vi "Autonomous Independent.vi"   [LabVIEW 2020]
doc: "This VI is called when autonomous begins, and will automatically be terminated when autonomous ends. You can carry out timed or sensor driven robot movement independently without needing to return to the caller."
uses:
  <vilib>/Rock Robotics/WPI/Utilities/WPI_GetSetVariantRefNum.vi
  <vilib>/Rock Robotics/Network Tables/NT Read String.vi
  <vilib>/Rock Robotics/Network Tables/NT Write Numeric Array.vi
  Autonomous/AutoGlobals.vi
panel:
  # "Be sure to right-click and choose Data Operations>>Make Current Value default if you want to save the array values with the VI"
types:
  T1 = typedef "WPI_JoystickDevRef.ctl" = cluster{"Device":T2}
  T2 = typedef "WPI_JoystickDeviceEnum.ctl" = enum16{"USB 0", "USB 1", "USB 2", "USB 3", "USB 4", "USB 5"}
  T3 = typedef "Trajectory_Library.lvlib/TRAJECTORY.ctl" = cluster{"TotalTImeSecs":dbl, "States":T4[]}
  T4 = typedef "Trajectory_Library.lvlib/TRAJ_STATE.ctl" = cluster{"TimeSeconds":dbl, "Velocity":dbl, "Acceleration":dbl, "POSE":T5, "Curvature":dbl}
  T5 = typedef "Trajectory_Library.lvlib/POSE2D.ctl" = cluster{"TRANSLATION":T6, "ROTATION":T7}
  T6 = typedef "Trajectory_Library.lvlib/TRANSLATION2D.ctl" = cluster{"X":dbl, "Y":dbl}
  T7 = typedef "Trajectory_Library.lvlib/ROTATION2D.ctl" = cluster{"VALUE":dbl, "COS":dbl, "SIN":dbl}
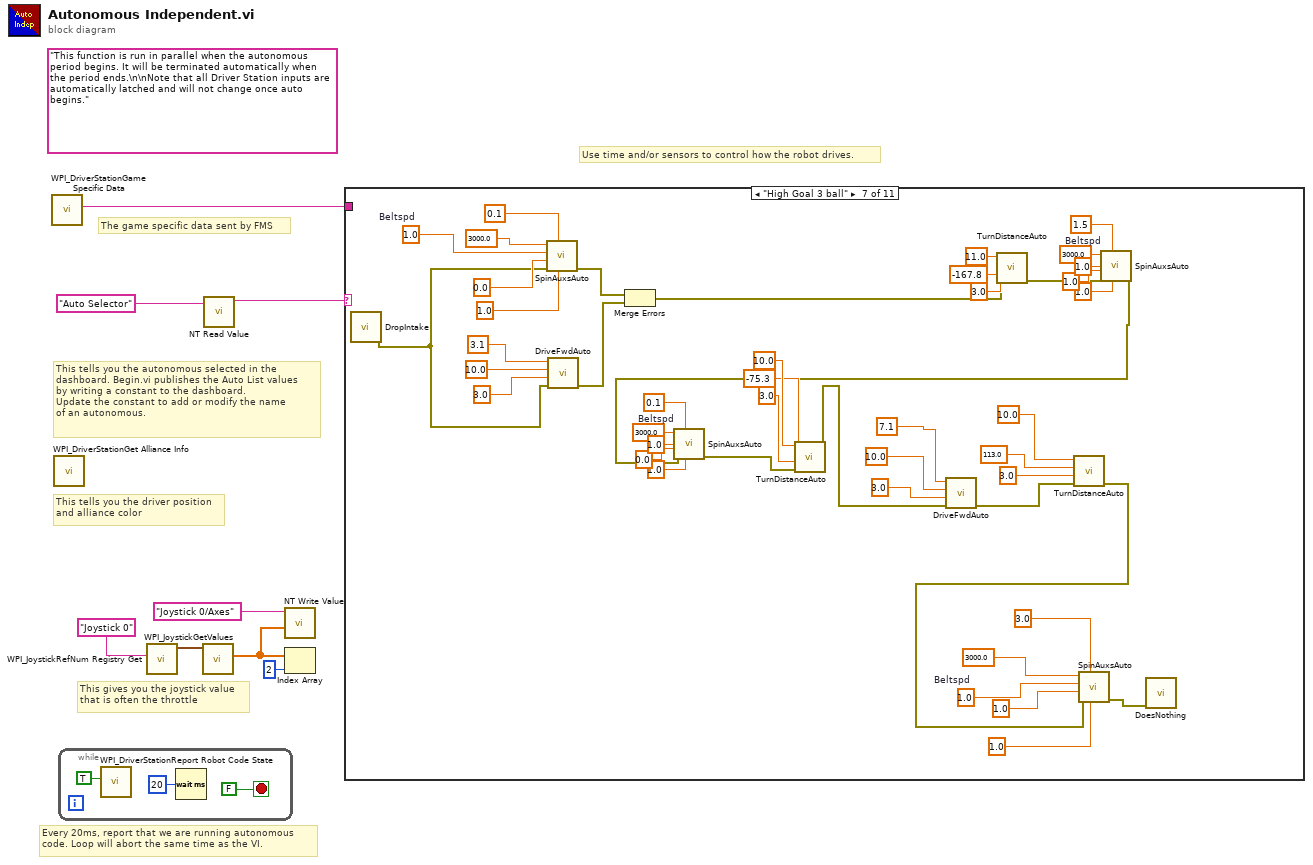
[diagram p0: block diagram]
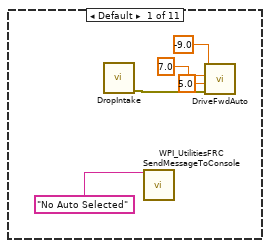
[diagram p2: hidden frame]
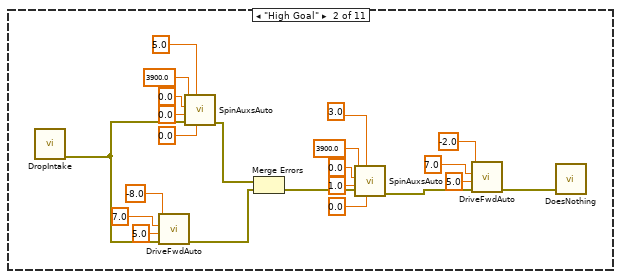
[diagram p3: hidden frame]
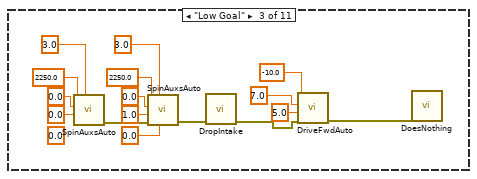
[diagram p4: hidden frame]
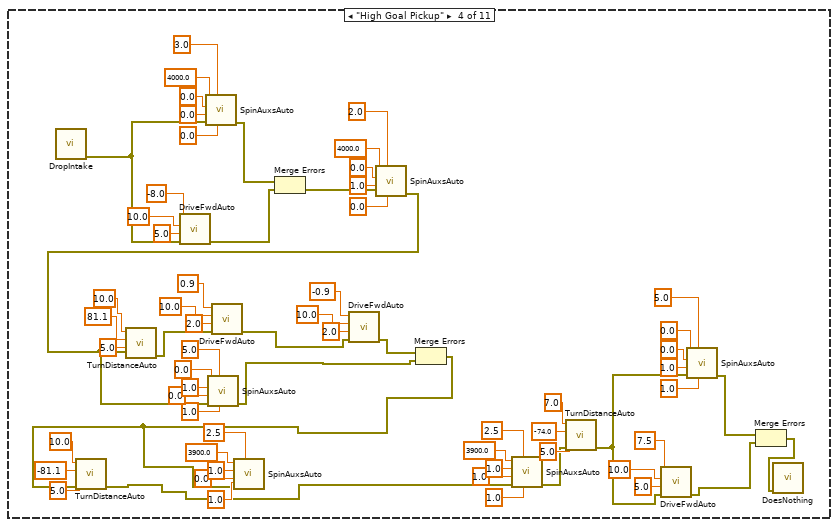
[diagram p5: hidden frame]
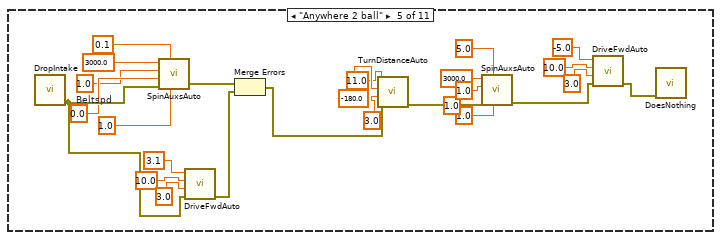
[diagram p6: hidden frame]
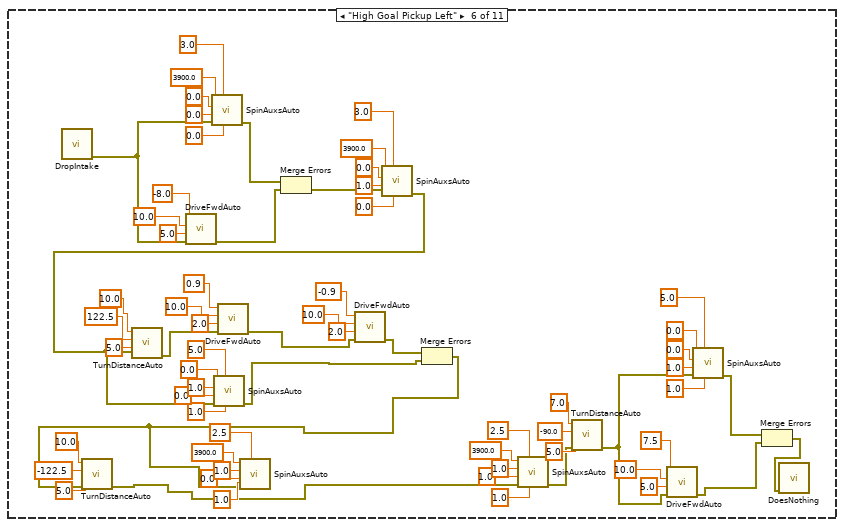
[diagram p7: hidden frame]
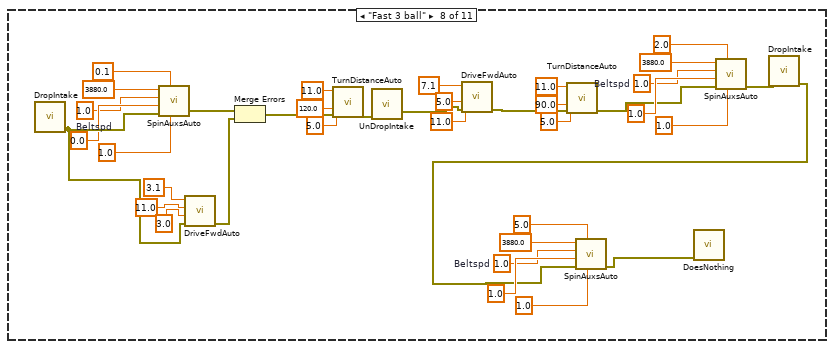
[diagram p8: hidden frame]
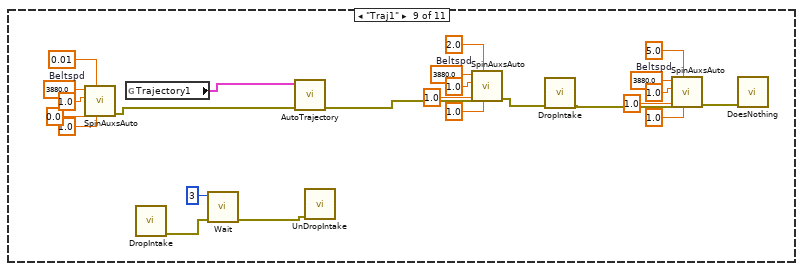
[diagram p9: hidden frame]
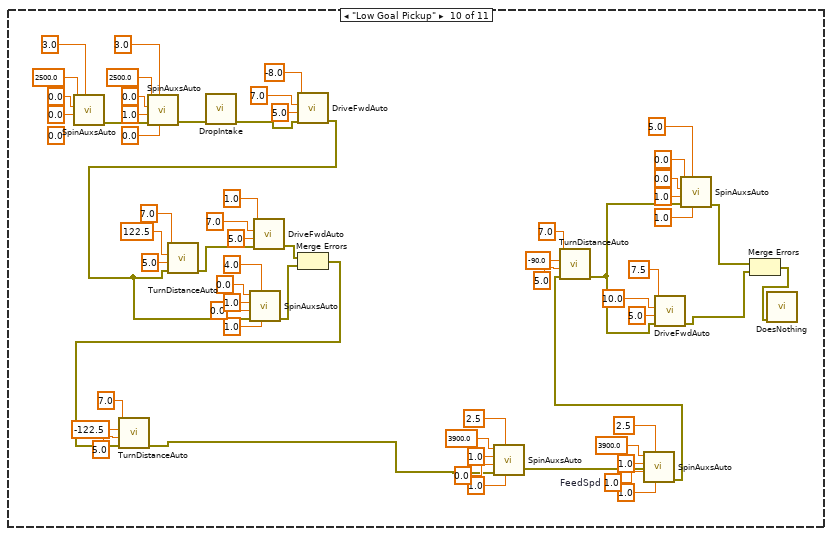
[diagram p10: hidden frame]
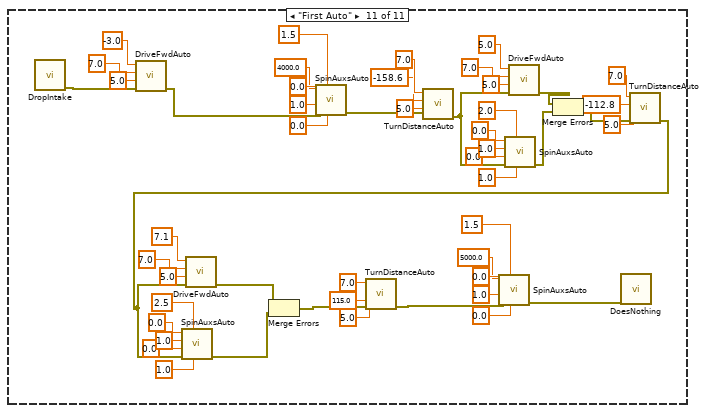
[diagram p11: hidden frame]
diagram:
  (unwired) "This function is run in parallel when the autonomous period begins. It will be terminated automatically when the period ends.\n\nNote that all Driver Station inputs are automatically latched and will not change once auto begins."
  # "The game specific data sent by FMS"
  # "This tells you the autonomous selected in the \ndashboard. Begin.vi publishes the Auto List values\nby writing a constant to the dashboard.\nUpdate the constant to add or modify the name\nof an autonomous."
  # "Every 20ms, report that we are running autonomous\ncode. Loop will abort the same time as the VI."
  # "This gives you the joystick value\nthat is often the throttle"
  # "Use time and/or sensors to control how the robot drives."
  # "This tells you the driver position\nand alliance color"
  n1 = call <vilib>:"WPI_DriverStationGame Specific Data.vi"() -> ("Game Specific Data"=w1:string)  [unwired: 11 in]
  n2 = call <vilib>:"WPI_DriverStationGet Alliance Info.vi"() -> ()  [unwired: 12 out]
  n3 = while {
    stop <- FALSE stop-if-true
    n4 = call <vilib>:"WPI_DriverStationReport Robot Code State.vi"("Autonomous"=TRUE) -> ()  [unwired: 10 in, 1 out]
    n5 = Wait (ms)(milliseconds to wait=u32 20) -> ()  [unwired: 1 out]
  }
  n6 = call <vilib>:"WPI_JoystickRefNum Registry Get.vi"("refnum name"="Joystick 0") -> ("JoystickDevRef"=w7:T1)  [unwired: 1 in, 9 out]
  n7 = call <vilib>:"WPI_JoystickGetValues.vi"("JoystickDevRef"=w7) -> ("Axes"=w3:dbl[])  [unwired: 6 in, 4 out]
  n8 = call-poly <vilib>:"NT Read Value.vi"("Name"="Auto Selector") -> ("String"=w4:string)  [unwired: 9 in, 1 out]
  n9 = call-poly <vilib>:"NT Write Value.vi"("Numeric Array"=w3, "Name"="Joystick 0/Axes") -> ()  [unwired: 9 in, 1 out]
  n10 = Index Array(array=w3, index=2) -> ()  [unwired: 1 out]
  n11 = case shown="\"High Goal 3 ball\"" w4 {
    tunnel: w1 -> [_ _ _ _ _ _ _ _ _ _ _]
    frame Default {
      n12 = call "DropIntake.vi"() -> ("error out"=w13:errorcluster)  [unwired: 11 in]
      n13 = call <vilib>:"WPI_UtilitiesFRC SendMessageToConsole.vi"("Message"="No Auto Selected") -> ()  [unwired: 14 in, 1 out]
      n14 = call "DriveFwdAuto.vi"("error in"=w13, "Timeout"=5.0, "MaxSpeed"=7.0, "Distance"=-9.0) -> ()  [unwired: 6 in, 2 out]
    }
    frame "High Goal" {
      n15 = call "DropIntake.vi"() -> ("error out"=w25:errorcluster)  [unwired: 11 in]
      n16 = call "DriveFwdAuto.vi"("error in"=w25, "Timeout"=5.0, "MaxSpeed"=7.0, "Distance"=-8.0) -> ("error out"=w23:errorcluster)  [unwired: 6 in, 1 out]
      n17 = call "SpinAuxsAuto.vi"("IntakeSpd"=0.0, "Time"=5.0, "error in"=w25, "FeedSpd"=0.0, "Beltspd"=0.0, "ShootSpd"=3900.0) -> ("error out"=w24:errorcluster)  [unwired: 4 in, 1 out]
      n18 = Merge Errors(w24, w23) -> (w22:errorcluster)
      n19 = call "SpinAuxsAuto.vi"("IntakeSpd"=0.0, "Time"=3.0, "error in"=w22, "FeedSpd"=1.0, "Beltspd"=0.0, "ShootSpd"=3900.0) -> ("error out"=w18:errorcluster)  [unwired: 4 in, 1 out]
      n20 = call "DriveFwdAuto.vi"("error in"=w18, "Timeout"=5.0, "MaxSpeed"=7.0, "Distance"=-2.0) -> ("error out"=w17:errorcluster)  [unwired: 6 in, 1 out]
      n21 = call "DoesNothing.vi"("error in (no error)"=w17) -> ()  [unwired: 10 in, 1 out]
    }
    frame "Low Goal" {
      (unwired) 0.0 ("IntakeSpd")
      n22 = call "SpinAuxsAuto.vi"("Time"=3.0, "FeedSpd"=0.0, "Beltspd"=0.0, "ShootSpd"=2250.0) -> ("error out"=w42:errorcluster)  [unwired: 6 in, 1 out]
      n23 = call "SpinAuxsAuto.vi"("IntakeSpd"=0.0, "Time"=3.0, "error in"=w42, "FeedSpd"=1.0, "Beltspd"=0.0, "ShootSpd"=2250.0) -> ("error out"=w41:errorcluster)  [unwired: 4 in, 1 out]
      n24 = call "DropIntake.vi"("error in"=w41) -> ("error out"=w40:errorcluster)  [unwired: 10 in]
      n25 = call "DriveFwdAuto.vi"("error in"=w40, "Timeout"=5.0, "MaxSpeed"=7.0, "Distance"=-10.0) -> ("error out"=w39:errorcluster)  [unwired: 6 in, 1 out]
      n26 = call "DoesNothing.vi"("error in (no error)"=w39) -> ()  [unwired: 10 in, 1 out]
    }
    frame "High Goal Pickup" {
      n27 = call "DropIntake.vi"() -> ("error out"=w118:errorcluster)  [unwired: 11 in]
      n28 = call "DriveFwdAuto.vi"("error in"=w118, "Timeout"=5.0, "MaxSpeed"=10.0, "Distance"=-8.0) -> ("error out"=w120:errorcluster)  [unwired: 6 in, 1 out]
      n29 = call "SpinAuxsAuto.vi"("IntakeSpd"=0.0, "Time"=3.0, "error in"=w118, "FeedSpd"=0.0, "Beltspd"=0.0, "ShootSpd"=4000.0) -> ("error out"=w119:errorcluster)  [unwired: 4 in, 1 out]
      n30 = Merge Errors(w119, w120) -> (w121:errorcluster)
      n31 = call "SpinAuxsAuto.vi"("IntakeSpd"=0.0, "Time"=2.0, "error in"=w121, "FeedSpd"=1.0, "Beltspd"=0.0, "ShootSpd"=4000.0) -> ("error out"=w84:errorcluster)  [unwired: 4 in, 1 out]
      n32 = call "TurnDistanceAuto.vi"("error in"=w84, "Timeout"=5.0, "Degrees"=81.1, "MaxSpeed"=10.0) -> ("error out"=w102:errorcluster)  [unwired: 6 in, 1 out]
      n33 = call "SpinAuxsAuto.vi"("IntakeSpd"=1.0, "Time"=5.0, "error in"=w84, "FeedSpd"=0.0, "Beltspd"=1.0, "ShootSpd"=0.0) -> ("error out"=w79:errorcluster)  [unwired: 4 in, 1 out]
      n34 = call "DriveFwdAuto.vi"("error in"=w102, "Timeout"=2.0, "MaxSpeed"=10.0, "Distance"=0.9) -> ("error out"=w80:errorcluster)  [unwired: 6 in, 1 out]
      n35 = call "DriveFwdAuto.vi"("error in"=w80, "Timeout"=2.0, "MaxSpeed"=10.0, "Distance"=-0.9) -> ("error out"=w78:errorcluster)  [unwired: 6 in, 1 out]
      n36 = Merge Errors(w78, w79) -> (w55:errorcluster)
      n37 = call "TurnDistanceAuto.vi"("error in"=w55, "Timeout"=5.0, "Degrees"=-81.1, "MaxSpeed"=10.0) -> ("error out"=w56:errorcluster)  [unwired: 6 in, 1 out]
      n38 = call "SpinAuxsAuto.vi"("IntakeSpd"=1.0, "Time"=2.5, "error in"=w55, "FeedSpd"=0.0, "Beltspd"=1.0, "ShootSpd"=3900.0) -> ()  [unwired: 4 in, 2 out]
      n39 = call "SpinAuxsAuto.vi"("IntakeSpd"=1.0, "Time"=2.5, "error in"=w56, "FeedSpd"=1.0, "Beltspd"=1.0, "ShootSpd"=3900.0) -> ("error out"=w57:errorcluster)  [unwired: 4 in, 1 out]
      n40 = call "TurnDistanceAuto.vi"("error in"=w57, "Timeout"=5.0, "Degrees"=-74.0, "MaxSpeed"=7.0) -> ("error out"=w66:errorcluster)  [unwired: 6 in, 1 out]
      n41 = call "DriveFwdAuto.vi"("error in"=w66, "Timeout"=5.0, "MaxSpeed"=10.0, "Distance"=7.5) -> ("error out"=w65:errorcluster)  [unwired: 6 in, 1 out]
      n42 = call "SpinAuxsAuto.vi"("IntakeSpd"=1.0, "Time"=5.0, "error in"=w66, "FeedSpd"=1.0, "Beltspd"=0.0, "ShootSpd"=0.0) -> ("error out"=w74:errorcluster)  [unwired: 4 in, 1 out]
      n43 = Merge Errors(w74, w65) -> (w64:errorcluster)
      n44 = call "DoesNothing.vi"("error in (no error)"=w64) -> ()  [unwired: 10 in, 1 out]
    }
    frame "Anywhere 2 ball" {
      w138 = 1.0  # Beltspd
      n45 = call "DropIntake.vi"() -> ("error out"=w145:errorcluster)  [unwired: 11 in]
      n46 = call "SpinAuxsAuto.vi"("IntakeSpd"=1.0, "Time"=0.1, "error in"=w145, "FeedSpd"=0.0, "Beltspd"=w138, "ShootSpd"=3000.0) -> ("error out"=w147:errorcluster)  [unwired: 4 in, 1 out]
      n47 = call "DriveFwdAuto.vi"("error in"=w145, "Timeout"=3.0, "MaxSpeed"=10.0, "Distance"=3.1) -> ("error out"=w146:errorcluster)  [unwired: 6 in, 1 out]
      n48 = Merge Errors(w147, w146) -> (w127:errorcluster)
      n49 = call "TurnDistanceAuto.vi"("error in"=w127, "Timeout"=3.0, "Degrees"=-180.0, "MaxSpeed"=11.0) -> ("error out"=w136:errorcluster)  [unwired: 6 in, 1 out]
      n50 = call "SpinAuxsAuto.vi"("IntakeSpd"=1.0, "Time"=5.0, "error in"=w136, "FeedSpd"=1.0, "Beltspd"=1.0, "ShootSpd"=3000.0) -> ("error out"=w123:errorcluster)  [unwired: 4 in, 1 out]
      n51 = call "DriveFwdAuto.vi"("error in"=w123, "Timeout"=3.0, "MaxSpeed"=10.0, "Distance"=-5.0) -> ("error out"=w122:errorcluster)  [unwired: 6 in, 1 out]
      n52 = call "DoesNothing.vi"("error in (no error)"=w122) -> ()  [unwired: 10 in, 1 out]
    }
    frame "High Goal Pickup Left" {
      n53 = call "DropIntake.vi"() -> ("error out"=w211:errorcluster)  [unwired: 11 in]
      n54 = call "DriveFwdAuto.vi"("error in"=w211, "Timeout"=5.0, "MaxSpeed"=10.0, "Distance"=-8.0) -> ("error out"=w213:errorcluster)  [unwired: 6 in, 1 out]
      n55 = call "SpinAuxsAuto.vi"("IntakeSpd"=0.0, "Time"=3.0, "error in"=w211, "FeedSpd"=0.0, "Beltspd"=0.0, "ShootSpd"=3900.0) -> ("error out"=w212:errorcluster)  [unwired: 4 in, 1 out]
      n56 = Merge Errors(w212, w213) -> (w214:errorcluster)
      n57 = call "SpinAuxsAuto.vi"("IntakeSpd"=0.0, "Time"=3.0, "error in"=w214, "FeedSpd"=1.0, "Beltspd"=0.0, "ShootSpd"=3900.0) -> ("error out"=w177:errorcluster)  [unwired: 4 in, 1 out]
      n58 = call "TurnDistanceAuto.vi"("error in"=w177, "Timeout"=5.0, "Degrees"=122.5, "MaxSpeed"=10.0) -> ("error out"=w195:errorcluster)  [unwired: 6 in, 1 out]
      n59 = call "SpinAuxsAuto.vi"("IntakeSpd"=1.0, "Time"=5.0, "error in"=w177, "FeedSpd"=0.0, "Beltspd"=1.0, "ShootSpd"=0.0) -> ("error out"=w172:errorcluster)  [unwired: 4 in, 1 out]
      n60 = call "DriveFwdAuto.vi"("error in"=w195, "Timeout"=2.0, "MaxSpeed"=10.0, "Distance"=0.9) -> ("error out"=w173:errorcluster)  [unwired: 6 in, 1 out]
      n61 = call "DriveFwdAuto.vi"("error in"=w173, "Timeout"=2.0, "MaxSpeed"=10.0, "Distance"=-0.9) -> ("error out"=w171:errorcluster)  [unwired: 6 in, 1 out]
      n62 = Merge Errors(w171, w172) -> (w148:errorcluster)
      n63 = call "TurnDistanceAuto.vi"("error in"=w148, "Timeout"=5.0, "Degrees"=-122.5, "MaxSpeed"=10.0) -> ("error out"=w149:errorcluster)  [unwired: 6 in, 1 out]
      n64 = call "SpinAuxsAuto.vi"("IntakeSpd"=1.0, "Time"=2.5, "error in"=w148, "FeedSpd"=0.0, "Beltspd"=1.0, "ShootSpd"=3900.0) -> ()  [unwired: 4 in, 2 out]
      n65 = call "SpinAuxsAuto.vi"("IntakeSpd"=1.0, "Time"=2.5, "error in"=w149, "FeedSpd"=1.0, "Beltspd"=1.0, "ShootSpd"=3900.0) -> ("error out"=w150:errorcluster)  [unwired: 4 in, 1 out]
      n66 = call "TurnDistanceAuto.vi"("error in"=w150, "Timeout"=5.0, "Degrees"=-90.0, "MaxSpeed"=7.0) -> ("error out"=w159:errorcluster)  [unwired: 6 in, 1 out]
      n67 = call "DriveFwdAuto.vi"("error in"=w159, "Timeout"=5.0, "MaxSpeed"=10.0, "Distance"=7.5) -> ("error out"=w158:errorcluster)  [unwired: 6 in, 1 out]
      n68 = call "SpinAuxsAuto.vi"("IntakeSpd"=1.0, "Time"=5.0, "error in"=w159, "FeedSpd"=1.0, "Beltspd"=0.0, "ShootSpd"=0.0) -> ("error out"=w167:errorcluster)  [unwired: 4 in, 1 out]
      n69 = Merge Errors(w167, w158) -> (w157:errorcluster)
      n70 = call "DoesNothing.vi"("error in (no error)"=w157) -> ()  [unwired: 10 in, 1 out]
    }
    frame "High Goal 3 ball" {
      w226 = 1.0  # Beltspd
      w232 = 1.0  # Beltspd
      w248 = 1.0  # Beltspd
      w253 = 1.0  # Beltspd
      n71 = call "DropIntake.vi"() -> ("error out"=w219:errorcluster)  [unwired: 11 in]
      n72 = call "SpinAuxsAuto.vi"("IntakeSpd"=1.0, "Time"=0.1, "error in"=w219, "FeedSpd"=0.0, "Beltspd"=w253, "ShootSpd"=3000.0) -> ("error out"=w216:errorcluster)  [unwired: 4 in, 1 out]
      n73 = call "DriveFwdAuto.vi"("error in"=w219, "Timeout"=3.0, "MaxSpeed"=10.0, "Distance"=3.1) -> ("error out"=w217:errorcluster)  [unwired: 6 in, 1 out]
      n74 = Merge Errors(w216, w217) -> (w218:errorcluster)
      n75 = call "TurnDistanceAuto.vi"("error in"=w218, "Timeout"=3.0, "Degrees"=-167.8, "MaxSpeed"=11.0) -> ("error out"=w244:errorcluster)  [unwired: 6 in, 1 out]
      n76 = call "SpinAuxsAuto.vi"("IntakeSpd"=1.0, "Time"=1.5, "error in"=w244, "FeedSpd"=1.0, "Beltspd"=w248, "ShootSpd"=3000.0) -> ("error out"=w222:errorcluster)  [unwired: 4 in, 1 out]
      n77 = call "SpinAuxsAuto.vi"("IntakeSpd"=1.0, "Time"=0.1, "error in"=w222, "FeedSpd"=0.0, "Beltspd"=w226, "ShootSpd"=3000.0) -> ("error out"=w221:errorcluster)  [unwired: 4 in, 1 out]
      n78 = call "TurnDistanceAuto.vi"("error in"=w221, "Timeout"=3.0, "Degrees"=-75.3, "MaxSpeed"=10.0) -> ("error out"=w238:errorcluster)  [unwired: 6 in, 1 out]
      n79 = call "DriveFwdAuto.vi"("error in"=w238, "Timeout"=3.0, "MaxSpeed"=10.0, "Distance"=7.1) -> ("error out"=w234:errorcluster)  [unwired: 6 in, 1 out]
      n80 = call "TurnDistanceAuto.vi"("error in"=w234, "Timeout"=3.0, "Degrees"=113.0, "MaxSpeed"=10.0) -> ("error out"=w220:errorcluster)  [unwired: 6 in, 1 out]
      n81 = call "SpinAuxsAuto.vi"("IntakeSpd"=1.0, "Time"=3.0, "error in"=w220, "FeedSpd"=1.0, "Beltspd"=w232, "ShootSpd"=3000.0) -> ("error out"=w228:errorcluster)  [unwired: 4 in, 1 out]
      n82 = call "DoesNothing.vi"("error in (no error)"=w228) -> ()  [unwired: 10 in, 1 out]
    }
    frame "Fast 3 ball" {
      w264 = 1.0  # Beltspd
      w271 = 1.0  # Beltspd
      w289 = 1.0  # Beltspd
      n83 = call "DropIntake.vi"() -> ("error out"=w296:errorcluster)  [unwired: 11 in]
      n84 = call "SpinAuxsAuto.vi"("IntakeSpd"=1.0, "Time"=0.1, "error in"=w296, "FeedSpd"=0.0, "Beltspd"=w289, "ShootSpd"=3880.0) -> ("error out"=w298:errorcluster)  [unwired: 4 in, 1 out]
      n85 = call "DriveFwdAuto.vi"("error in"=w296, "Timeout"=3.0, "MaxSpeed"=11.0, "Distance"=3.1) -> ("error out"=w297:errorcluster)  [unwired: 6 in, 1 out]
      n86 = Merge Errors(w298, w297) -> (w287:errorcluster)
      n87 = call "TurnDistanceAuto.vi"("error in"=w287, "Timeout"=5.0, "Degrees"=120.0, "MaxSpeed"=11.0) -> ("error out"=w276:errorcluster)  [unwired: 6 in, 1 out]
      n88 = call "UnDropIntake.vi"("error in"=w276) -> ("error out"=w275:errorcluster)  [unwired: 10 in]
      n89 = call "DriveFwdAuto.vi"("error in"=w275, "Timeout"=5.0, "MaxSpeed"=11.0, "Distance"=7.1) -> ("error out"=w277:errorcluster)  [unwired: 6 in, 1 out]
      n90 = call "TurnDistanceAuto.vi"("error in"=w277, "Timeout"=5.0, "Degrees"=90.0, "MaxSpeed"=11.0) -> ("error out"=w269:errorcluster)  [unwired: 6 in, 1 out]
      n91 = call "SpinAuxsAuto.vi"("IntakeSpd"=1.0, "Time"=2.0, "error in"=w269, "FeedSpd"=1.0, "Beltspd"=w271, "ShootSpd"=3880.0) -> ("error out"=w268:errorcluster)  [unwired: 4 in, 1 out]
      n92 = call "DropIntake.vi"("error in"=w268) -> ("error out"=w262:errorcluster)  [unwired: 10 in]
      n93 = call "SpinAuxsAuto.vi"("IntakeSpd"=1.0, "Time"=5.0, "error in"=w262, "FeedSpd"=1.0, "Beltspd"=w264, "ShootSpd"=3880.0) -> ("error out"=w261:errorcluster)  [unwired: 4 in, 1 out]
      n94 = call "DoesNothing.vi"("error in (no error)"=w261) -> ()  [unwired: 10 in, 1 out]
    }
    frame "Traj1" {
      w302 = 1.0  # Beltspd
      w312 = 1.0  # Beltspd
      w318 = 1.0  # Beltspd
      n95 = call "SpinAuxsAuto.vi"("IntakeSpd"=1.0, "Time"=0.01, "FeedSpd"=0.0, "Beltspd"=w312, "ShootSpd"=3880.0) -> ("error out"=w310:errorcluster)  [unwired: 5 in, 1 out]
      n96 = global read "AutoGlobals.vi" "Trajectory1"() -> (w322:T3)
      n97 = call "DropIntake.vi"() -> ("error out"=w308:errorcluster)  [unwired: 11 in]
      n98 = call "Wait.vi"("SecondsWait"=u32 3, "error in"=w308) -> ("error out"=w309:errorcluster)  [unwired: 8 in]
      n99 = call "AutoTrajectory.vi"("error in"=w310, "Trajectory"=w322) -> ("error out"=w316:errorcluster)  [unwired: 6 in, 3 out]
      n100 = call "UnDropIntake.vi"("error in"=w309) -> ()  [unwired: 10 in, 1 out]
      n101 = call "SpinAuxsAuto.vi"("IntakeSpd"=1.0, "Time"=2.0, "error in"=w316, "FeedSpd"=1.0, "Beltspd"=w318, "ShootSpd"=3880.0) -> ("error out"=w306:errorcluster)  [unwired: 4 in, 1 out]
      n102 = call "DropIntake.vi"("error in"=w306) -> ("error out"=w300:errorcluster)  [unwired: 10 in]
      n103 = call "SpinAuxsAuto.vi"("IntakeSpd"=1.0, "Time"=5.0, "error in"=w300, "FeedSpd"=1.0, "Beltspd"=w302, "ShootSpd"=3880.0) -> ("error out"=w299:errorcluster)  [unwired: 4 in, 1 out]
      n104 = call "DoesNothing.vi"("error in (no error)"=w299) -> ()  [unwired: 10 in, 1 out]
    }
    frame "Low Goal Pickup" {
      w328 = 1.0  # FeedSpd
      (unwired) 0.0 ("IntakeSpd")
      n105 = call "SpinAuxsAuto.vi"("Time"=3.0, "FeedSpd"=0.0, "Beltspd"=0.0, "ShootSpd"=2500.0) -> ("error out"=w382:errorcluster)  [unwired: 6 in, 1 out]
      n106 = call "SpinAuxsAuto.vi"("IntakeSpd"=0.0, "Time"=3.0, "error in"=w382, "FeedSpd"=1.0, "Beltspd"=0.0, "ShootSpd"=2500.0) -> ("error out"=w383:errorcluster)  [unwired: 4 in, 1 out]
      n107 = call "DropIntake.vi"("error in"=w383) -> ("error out"=w384:errorcluster)  [unwired: 10 in]
      n108 = call "DriveFwdAuto.vi"("error in"=w384, "Timeout"=5.0, "MaxSpeed"=7.0, "Distance"=-8.0) -> ("error out"=w351:errorcluster)  [unwired: 6 in, 1 out]
      n109 = call "TurnDistanceAuto.vi"("error in"=w351, "Timeout"=5.0, "Degrees"=122.5, "MaxSpeed"=7.0) -> ("error out"=w366:errorcluster)  [unwired: 6 in, 1 out]
      n110 = call "SpinAuxsAuto.vi"("IntakeSpd"=1.0, "Time"=4.0, "error in"=w351, "FeedSpd"=0.0, "Beltspd"=1.0, "ShootSpd"=0.0) -> ("error out"=w367:errorcluster)  [unwired: 4 in, 1 out]
      n111 = call "DriveFwdAuto.vi"("error in"=w366, "Timeout"=5.0, "MaxSpeed"=7.0, "Distance"=1.0) -> ("error out"=w368:errorcluster)  [unwired: 6 in, 1 out]
      n112 = Merge Errors(w368, w367) -> (w369:errorcluster)
      n113 = call "TurnDistanceAuto.vi"("error in"=w369, "Timeout"=5.0, "Degrees"=-122.5, "MaxSpeed"=7.0) -> ("error out"=w330:errorcluster)  [unwired: 6 in, 1 out]
      n114 = call "SpinAuxsAuto.vi"("IntakeSpd"=1.0, "Time"=2.5, "error in"=w330, "FeedSpd"=0.0, "Beltspd"=1.0, "ShootSpd"=3900.0) -> ("error out"=w324:errorcluster)  [unwired: 4 in, 1 out]
      n115 = call "SpinAuxsAuto.vi"("IntakeSpd"=1.0, "Time"=2.5, "error in"=w324, "FeedSpd"=w328, "Beltspd"=1.0, "ShootSpd"=3900.0) -> ("error out"=w323:errorcluster)  [unwired: 4 in, 1 out]
      n116 = call "TurnDistanceAuto.vi"("error in"=w323, "Timeout"=5.0, "Degrees"=-90.0, "MaxSpeed"=7.0) -> ("error out"=w348:errorcluster)  [unwired: 6 in, 1 out]
      n117 = call "DriveFwdAuto.vi"("error in"=w348, "Timeout"=5.0, "MaxSpeed"=10.0, "Distance"=7.5) -> ("error out"=w349:errorcluster)  [unwired: 6 in, 1 out]
      n118 = call "SpinAuxsAuto.vi"("IntakeSpd"=1.0, "Time"=5.0, "error in"=w348, "FeedSpd"=1.0, "Beltspd"=0.0, "ShootSpd"=0.0) -> ("error out"=w347:errorcluster)  [unwired: 4 in, 1 out]
      n119 = Merge Errors(w347, w349) -> (w350:errorcluster)
      n120 = call "DoesNothing.vi"("error in (no error)"=w350) -> ()  [unwired: 10 in, 1 out]
    }
    frame "First Auto" {
      n121 = call "DropIntake.vi"() -> ("error out"=w386:errorcluster)  [unwired: 11 in]
      n122 = call "DriveFwdAuto.vi"("error in"=w386, "Timeout"=5.0, "MaxSpeed"=7.0, "Distance"=-3.0) -> ("error out"=w385:errorcluster)  [unwired: 6 in, 1 out]
      n123 = call "SpinAuxsAuto.vi"("IntakeSpd"=0.0, "Time"=1.5, "error in"=w385, "FeedSpd"=1.0, "Beltspd"=0.0, "ShootSpd"=4000.0) -> ("error out"=w430:errorcluster)  [unwired: 4 in, 1 out]
      n124 = call "TurnDistanceAuto.vi"("error in"=w430, "Timeout"=5.0, "Degrees"=-158.6, "MaxSpeed"=7.0) -> ("error out"=w426:errorcluster)  [unwired: 6 in, 1 out]
      n125 = call "SpinAuxsAuto.vi"("IntakeSpd"=1.0, "Time"=2.0, "error in"=w426, "FeedSpd"=0.0, "Beltspd"=1.0, "ShootSpd"=0.0) -> ("error out"=w425:errorcluster)  [unwired: 4 in, 1 out]
      n126 = call "DriveFwdAuto.vi"("error in"=w426, "Timeout"=5.0, "MaxSpeed"=7.0, "Distance"=5.0) -> ("error out"=w424:errorcluster)  [unwired: 6 in, 1 out]
      n127 = Merge Errors(w424, w425) -> (w415:errorcluster)
      n128 = call "TurnDistanceAuto.vi"("error in"=w415, "Timeout"=5.0, "Degrees"=-112.8, "MaxSpeed"=7.0) -> ("error out"=w401:errorcluster)  [unwired: 6 in, 1 out]
      n129 = call "SpinAuxsAuto.vi"("IntakeSpd"=1.0, "Time"=2.5, "error in"=w401, "FeedSpd"=0.0, "Beltspd"=1.0, "ShootSpd"=0.0) -> ("error out"=w411:errorcluster)  [unwired: 4 in, 1 out]
      n130 = call "DriveFwdAuto.vi"("error in"=w401, "Timeout"=5.0, "MaxSpeed"=7.0, "Distance"=7.1) -> ("error out"=w410:errorcluster)  [unwired: 6 in, 1 out]
      n131 = Merge Errors(w410, w411) -> (w400:errorcluster)
      n132 = call "TurnDistanceAuto.vi"("error in"=w400, "Timeout"=5.0, "Degrees"=115.0, "MaxSpeed"=7.0) -> ("error out"=w391:errorcluster)  [unwired: 6 in, 1 out]
      n133 = call "SpinAuxsAuto.vi"("IntakeSpd"=0.0, "Time"=1.5, "error in"=w391, "FeedSpd"=1.0, "Beltspd"=0.0, "ShootSpd"=5000.0) -> ("error out"=w390:errorcluster)  [unwired: 4 in, 1 out]
      n134 = call "DoesNothing.vi"("error in (no error)"=w390) -> ()  [unwired: 10 in, 1 out]
    }
  }
